vi "Render.vi"(8 "error in (no error)":errorcluster, 10 "String in":string, 11 "Blockquote in":refnum<class "Blockquote.lvclass">) -> (0 "error out":errorcluster, 2 "String out":string, 3 "Blockquote out":refnum<class "Blockquote.lvclass">)   [LabVIEW 2021, in "Markdown.lvlib" / "Blockquote.lvclass"]
uses:
  Blockquote.lvclass
  C:/GitHub/Markdown/src/Markdown/Markdown.lvclass
  GetBlockquoteTag.vi
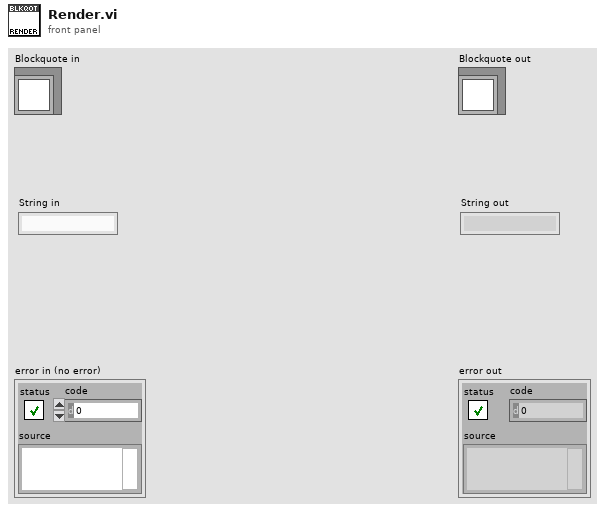
[diagram p1: front panel]
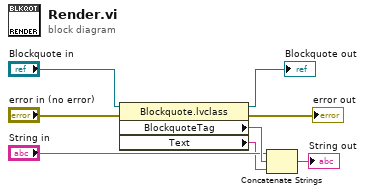
[diagram p0: block diagram]
diagram:
  n1 = property class="Blockquote.lvclass"(reference="Blockquote in", error in="error in (no error)") -> (reference out=→"Blockquote out":refnum<class "Blockquote.lvclass">, error out=→"error out":errorcluster, "BlockquoteTag"=w6:string, "Text"=w3:string)
  n2 = Concatenate Strings("String in", w6, w3) -> (→"String out":string)
